vi "archivoaespectro.vi"(5 "data 2":string[][](array[string])) -> (3 "opciones":bool[](array[boolean]), 4 "Control de espejos 3":T5={"Movimiento de spot en y"=0.78, "Movimiento de spot en x"=0.5255, "tipo "=enum."barrido", "yFin"=0.82, "Paso"=0.01, "xFin"=0.5655} {"Movimiento de spot en x" scale=-10.0..10.0; "Movimiento de spot en y" min=-10.0 max=10.0 scale=-10.0..10.0}, 6 "config. Polarizador 2":T4={"pos inic"=0.0, "pos.final"=5.0, "incremento"=1.0, "velocidad"=0.0}, 8 "Config. fotodiodo y potenciometro 2":T2={"tiempo. lect."=300, "num. med"=20, "tiempo. lectura"=0, "average rate"=0, "Readout Config"="POW", "Tipo de Medición"=enum."Lockin", "usar multimetro"=FALSE}, 10 "Config. voltaje y corriente 2":T3 {"Measurement Function (0:Voltage)" items=["Voltage", "Current", "Power"]; "Unit(V)" items=["V", "mV", "kV", "A", "mA"]; "Function(0:Voltage)" items=["Voltage", "Current"]}, 14 "orden":T6(array[ring]), 15 "Control CCD 2":T1={"Numero de lecturas"=0, "tiempo de lectura (ms)"=100, "Exposure"=0.053229, "Valor Gamma"=1.0, "Ganancia"=33, "Opción"=enum."Espectro", "VISA resource name"="", "Enable Strobe (Disabled)"=FALSE} {"Ganancia" min=0 max=100; "Valor Gamma" min=1.0 max=2.2; "Exposure" min=5e-05 max=0.053229})   [LabVIEW 2016]
panel:
  in  "Control CCD":T1={"Numero de lecturas"=0, "tiempo de lectura (ms)"=100, "Exposure"=0.053229, "Valor Gamma"=1.0, "Ganancia"=33, "Opción"=enum."Espectro", "VISA resource name"="", "Enable Strobe (Disabled)"=FALSE} {"Ganancia" min=0 max=100; "Valor Gamma" min=1.0 max=2.2; "Exposure" min=5e-05 max=0.053229}
  in  "Config. fotodiodo y potenciometro":T2={"tiempo. lect."=300, "num. med"=20, "tiempo. lectura"=0, "average rate"=0, "Readout Config"="POW", "Tipo de Medición"=enum."Lockin", "usar multimetro"=FALSE}
  in  "Config. voltaje y corriente":T3 {"Measurement Function (0:Voltage)" items=["Voltage", "Current", "Power"]; "Unit(V)" items=["V", "mV", "kV", "A", "mA"]; "Function(0:Voltage)" items=["Voltage", "Current"]}
  in  "config. Polarizador":T4={"pos inic"=0.0, "pos.final"=5.0, "incremento"=1.0, "velocidad"=0.0}
  in  "Control de espejos 2":T5={"Movimiento de spot en y"=0.78, "Movimiento de spot en x"=0.5255, "tipo "=enum."barrido", "yFin"=0.82, "Paso"=0.01, "xFin"=0.5655} {"Movimiento de spot en x" scale=-10.0..10.0; "Movimiento de spot en y" min=-10.0 max=10.0 scale=-10.0..10.0}
  in  "Array":bool[](array[boolean])=[FALSE, FALSE, FALSE, FALSE, FALSE]
  # "Espectro"
  # "Imágen"
  # "Espectro"
  # "Imágen"
  # "Amplificador Lock in"
  # "potenciometro"
  # "Amplificador Lock in"
  # "potenciometro"
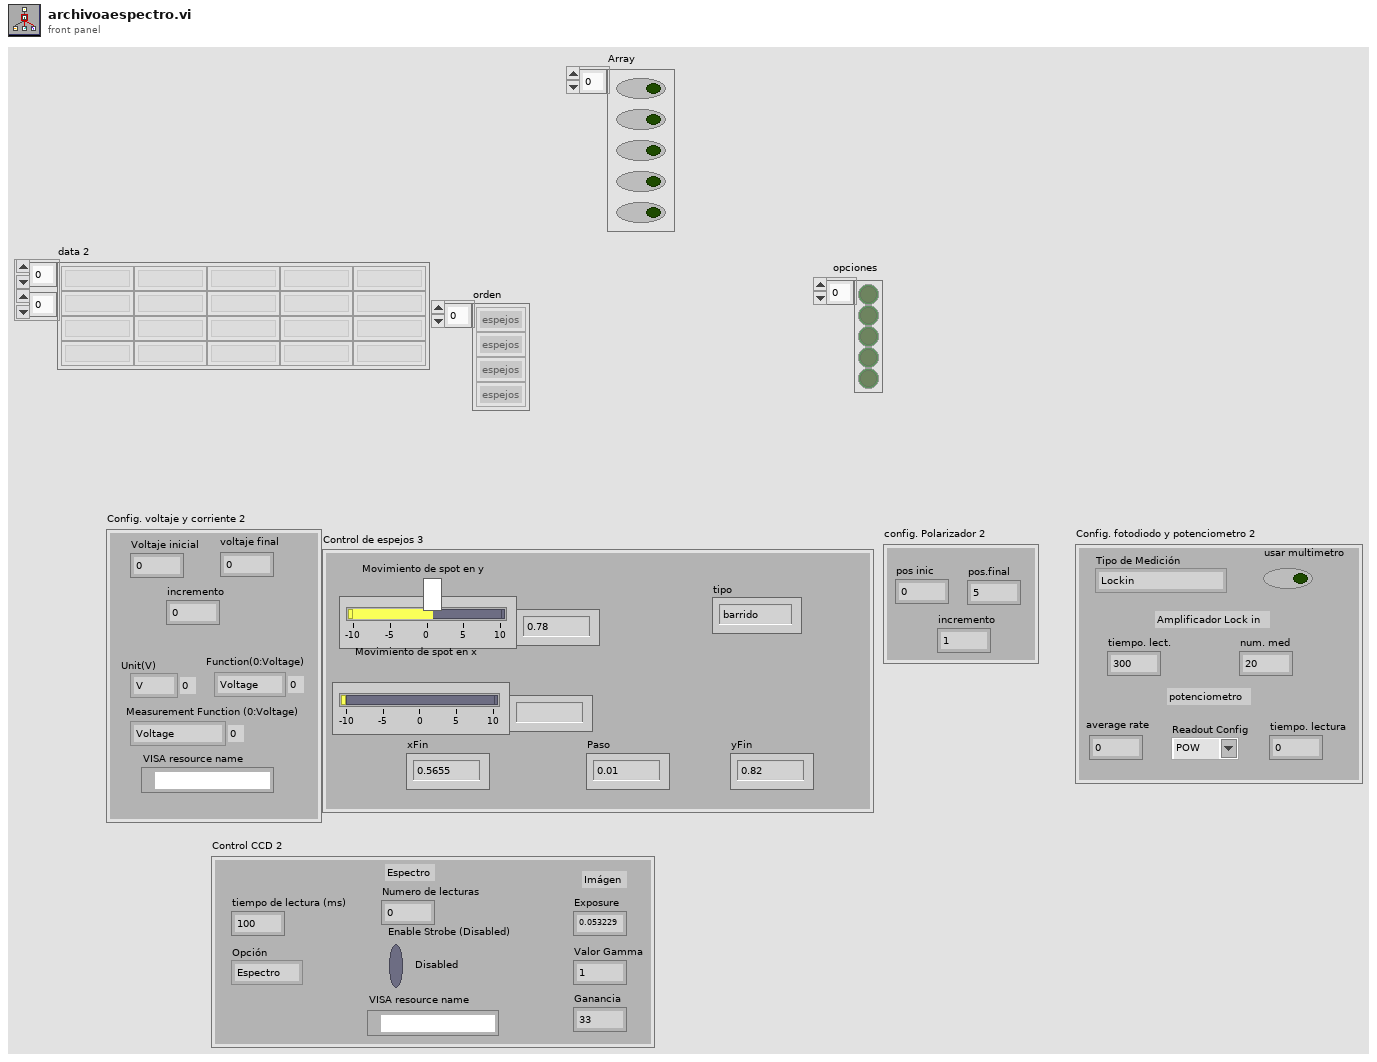
[diagram p1: front panel]
types:
  T1 = cluster{"Numero de lecturas":i32, "tiempo de lectura (ms)":u32, "Exposure":dbl, "Valor Gamma":dbl, "Ganancia":i64, "Opción":enum16{"Espectro", "Imágen"}, "VISA resource name":refnum<visa-resource-name>, "Enable Strobe (Disabled)":bool}
  T2 = cluster{"tiempo. lect.":i32, "num. med":i32, "tiempo. lectura":i32, "average rate":i32, "Readout Config":string, "Tipo de Medición":enum16{"Lockin", "Lockin-potenciometro", "Potenciometro"}, "usar multimetro":bool}
  T3 = cluster{"Voltaje inicial":dbl, "incremento":dbl, " voltaje final":dbl, "Function(0:Voltage)":u16, "Unit(V)":u16, "Measurement Function (0:Voltage)":u16, "VISA resource name":refnum<visa-resource-name>}
  T4 = cluster{"pos inic":dbl, "pos.final":dbl, "incremento":dbl, "velocidad":dbl}
  T5 = cluster{"Movimiento de spot en y":dbl, "Movimiento de spot en x":ext, "tipo ":enum16{"manual", "barrido"}, "yFin":dbl, "Paso":dbl, "xFin":dbl}
  T6 = enum16{"espejos", "polarizador", "voltaje", "potenciometro y lockin", "CCD"}[]
  T7 = enum16{"espejos", "polarizador", "voltaje", "potenciometro y lockin", "CCD"}
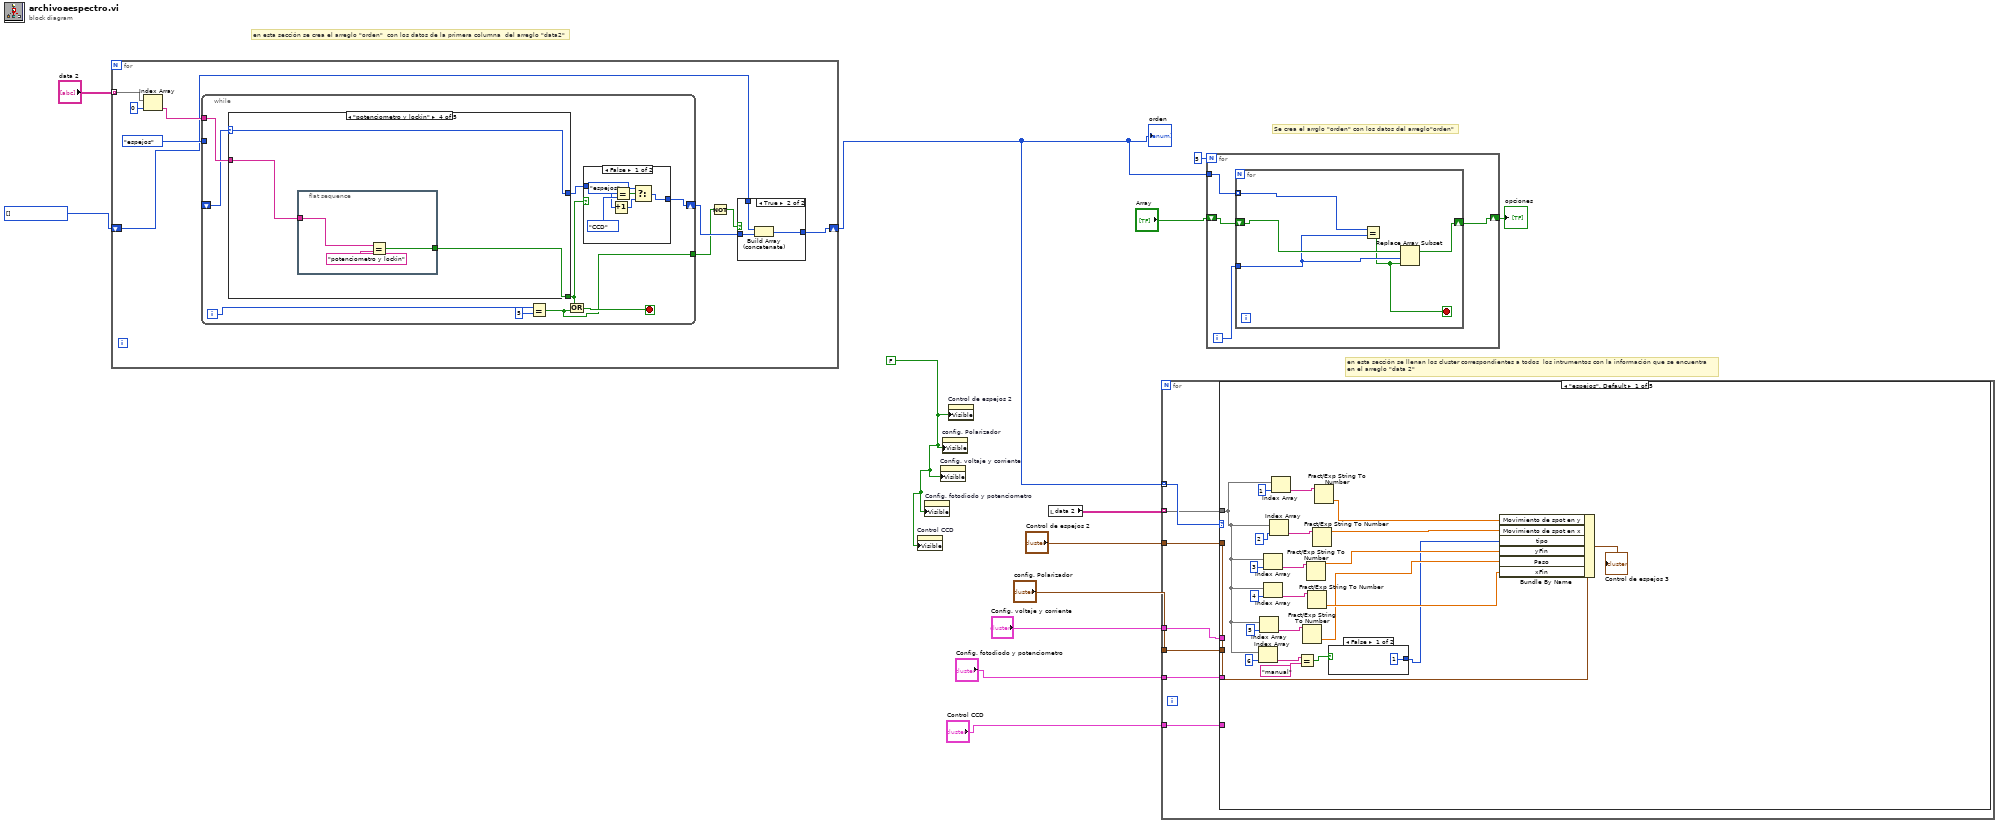
[diagram p0: block diagram]
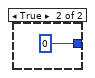
[diagram p2: hidden frame]
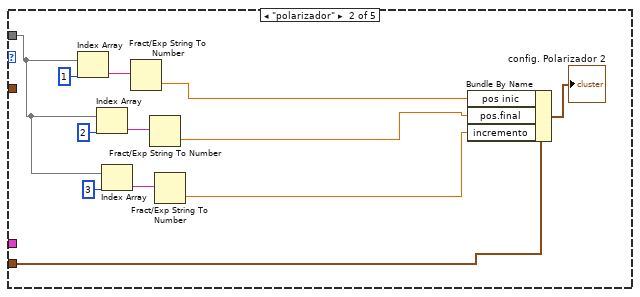
[diagram p3: hidden frame]
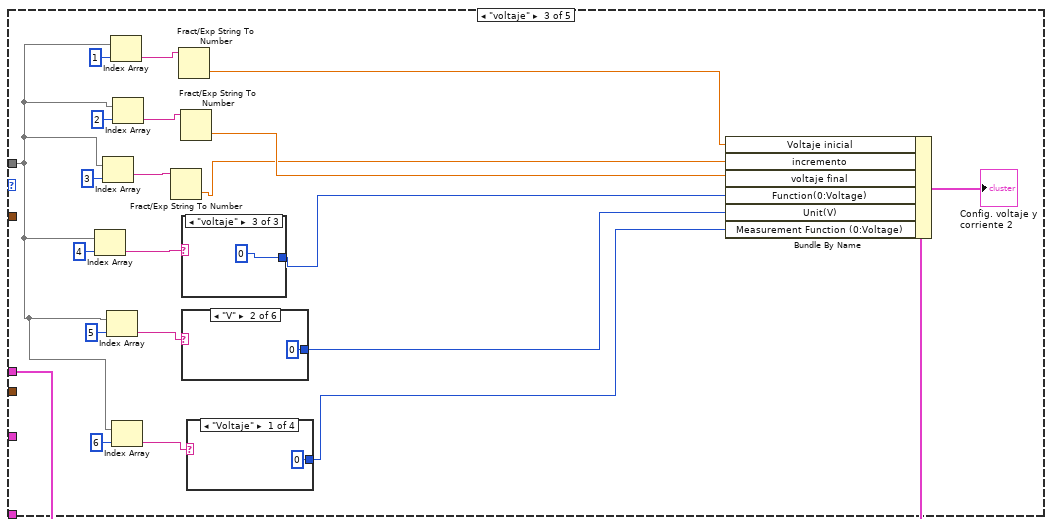
[diagram p4: hidden frame]
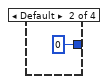
[diagram p5: hidden frame]
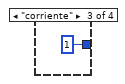
[diagram p6: hidden frame]
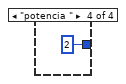
[diagram p7: hidden frame]
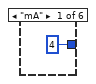
[diagram p8: hidden frame]
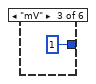
[diagram p9: hidden frame]
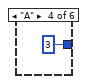
[diagram p10: hidden frame]
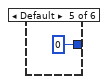
[diagram p11: hidden frame]
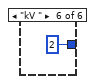
[diagram p12: hidden frame]
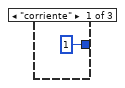
[diagram p13: hidden frame]
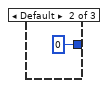
[diagram p14: hidden frame]
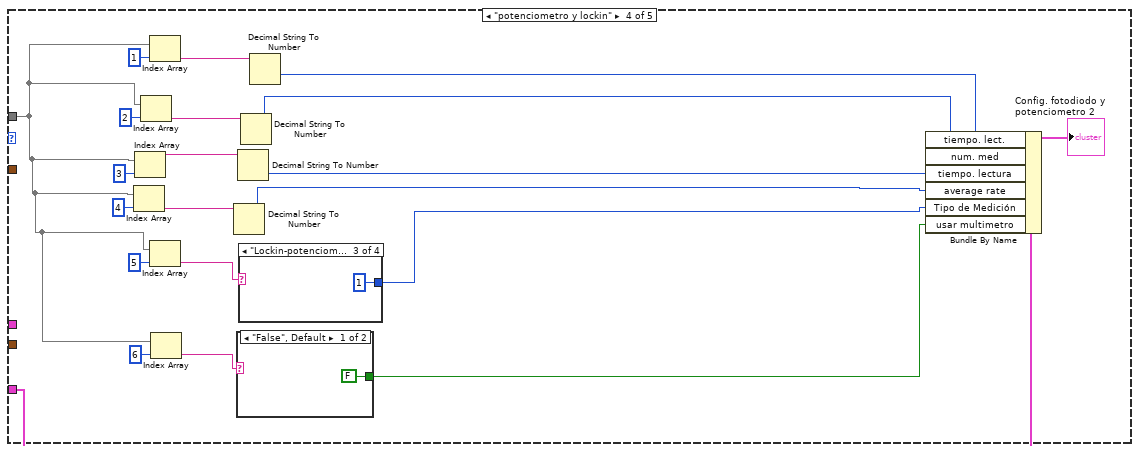
[diagram p15: hidden frame]
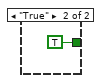
[diagram p16: hidden frame]
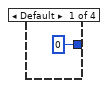
[diagram p17: hidden frame]
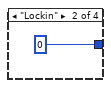
[diagram p18: hidden frame]
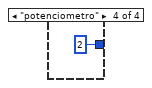
[diagram p19: hidden frame]
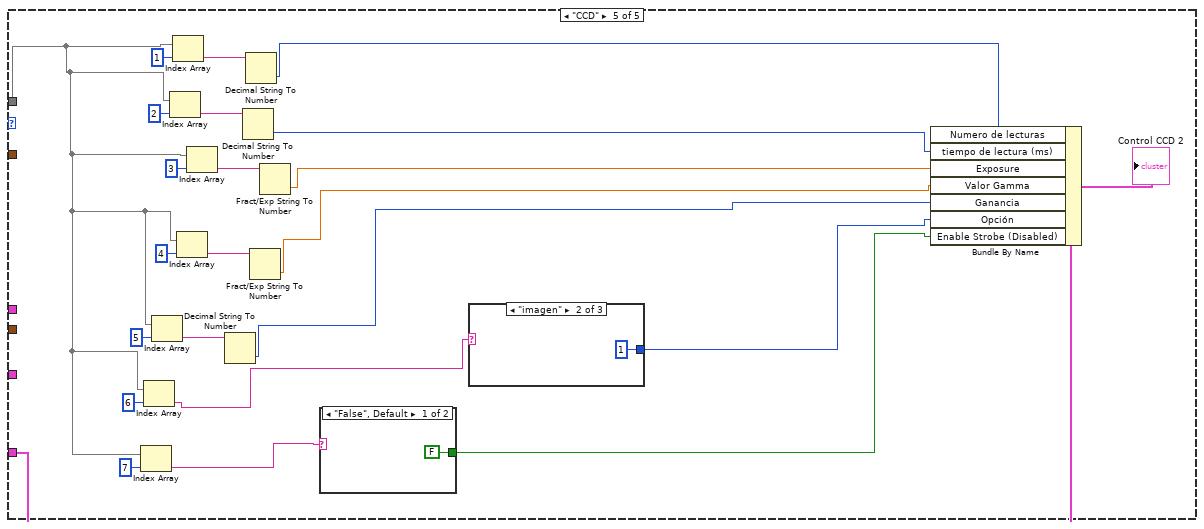
[diagram p20: hidden frame]
diagram:
  w1 = FALSE ("Visible")
  w9 = T6 [] items=["espejos", "polarizador", "voltaje", "potenciometro y lockin", "CCD"] ("Array 3")
  # "en esta sección se llenan los cluster correspondientes a todos  los intrumentos con la información que se encuentra\nen el arreglo \"data 2\""
  # "Se crea el arrglo \"orden\" con los datos del arreglo\"orden\""
  # "en esta sección se crea el arreglo \"orden\"  con los datos de la primera columna  del arreglo \"data2\""
  n1 = for {
    tunnel: "data 2" -> [w22] mode=indexing
    shift-right: [w14] -> w8
    shift-left: w9 -> [w15]
    n2 = Index Array(array=w22, index=0) -> (element=w20:string)
    n3 = while {
      tunnel: w20 -> [w35]
      tunnel: T7."espejos" ("Enum") -> [_]
      shift-right: [w30] -> w18
      shift-left: _ -> [w34]
      tunnel: [w27] -> w16
      i -> [w33]
      stop <- w31 stop-if-true
      n4 = case shown="\"potenciometro y lockin\"" w34 {
        selector: w34 -> [w43 w51 w57 w63 w69]
        tunnel: w35 -> [w45 w49 w56 w62 w68]
        tunnel: [w43 w51 w57 w63 w69] -> w28
        tunnel: [w44 w50 w55 w61 w67] -> w29
        frame "espejos", Default {
          n5 = flat-sequence {
            tunnel: w45 -> [w47]
            tunnel: [w46] -> w44
            frame #0 {
              n6 = Equal?(x=w47, y="espejos") -> (x = y?=w46:bool)
            }
          }
        }
        frame "polarizador" {
          n7 = flat-sequence {
            tunnel: w49 -> [w53]
            tunnel: [w52] -> w50
            frame #0 {
              n8 = Equal?(x=w53, y="polarizador") -> (x = y?=w52:bool)
            }
          }
        }
        frame "voltaje" {
          n9 = flat-sequence {
            tunnel: w56 -> [w59]
            tunnel: [w58] -> w55
            frame #0 {
              n10 = Equal?(x=w59, y="voltaje") -> (x = y?=w58:bool)
            }
          }
        }
        frame "potenciometro y lockin" {
          n11 = flat-sequence {
            tunnel: w62 -> [w65]
            tunnel: [w64] -> w61
            frame #0 {
              n12 = Equal?(x=w65, y="potenciometro y lockin") -> (x = y?=w64:bool)
            }
          }
        }
        frame "CCD" {
          n13 = flat-sequence {
            tunnel: w68 -> [w71]
            tunnel: [w70] -> w67
            frame #0 {
              n14 = Equal?(x=w71, y=" CCD") -> (x = y?=w70:bool)
            }
          }
        }
      }
      n15 = Equal?(x=w33, y=5) -> (x = y?=w27:bool)
      n16 = Or(x=w29, y=w27) -> (x .or. y?=w31:bool)
      n17 = case shown="False" w29 {
        tunnel: [w36 w42] -> w30
        tunnel: w28 -> [w38 w42]
        frame False {
          n18 = Increment(x=w38) -> (x+1=w39:T7)
          n19 = Equal?(x=w38, y=T7."CCD" ("x")) -> (x = y?=w41:bool)
          n20 = Select(t=T7."espejos", s=w41, f=w39) -> (s? t:f=w36:T7)
        }
        frame True {
        }
      }
    }
    n21 = Not(x=w16) -> (.not. x?=w17:bool)
    n22 = case shown="True" w17 {
      tunnel: w15 -> [w23 w26]
      tunnel: w18 -> [_ w25]
      tunnel: [w23 w24] -> w14
      frame False {
      }
      frame True {
        n23 = Build Array (concatenate)(w26, w25) -> (w24:T6)
      }
    }
  }
  "orden" <- w8
  n24 = property on="Control CCD" class="Clust (strict)"("Visible"=w1) -> ()  [unwired: 2 in, 2 out]
  n25 = property on="Config. fotodiodo y potenciometro" class="Clust (strict)"("Visible"=w1) -> ()  [unwired: 2 in, 2 out]
  n26 = property on="Config. voltaje y corriente" class="Clust (strict)"("Visible"=w1) -> ()  [unwired: 2 in, 2 out]
  n27 = property on="config. Polarizador" class="Clust (strict)"("Visible"=w1) -> ()  [unwired: 2 in, 2 out]
  n28 = property on="Control de espejos 2" class="Clust (strict)"("Visible"=w1) -> ()  [unwired: 2 in, 2 out]
  n29 = local read "data 2"() -> (w7:string[][])
  n30 = for {
    tunnel: w8 -> [w79] mode=indexing
    tunnel: w7 -> [w78] mode=indexing
    tunnel: "Control de espejos 2" -> [w77]
    tunnel: "config. Polarizador" -> [w76]
    tunnel: "Config. voltaje y corriente" -> [w75]
    tunnel: "Config. fotodiodo y potenciometro" -> [w74]
    tunnel: "Control CCD" -> [w73]
    n31 = case shown="\"espejos\", Default" w79 {
      tunnel: w78 -> [w86 w106 w118 w154 w184]
      tunnel: w77 -> [w101 _ _ _ _]
      tunnel: w76 -> [_ w115 _ _ _]
      tunnel: w75 -> [_ _ w136 _ _]
      tunnel: w74 -> [_ _ _ w170 _]
      tunnel: w73 -> [_ _ _ _ w200]
      frame "espejos", Default {
        n32 = Index Array(array=w86, index=6) -> (element=w84:string)
        n33 = Index Array(array=w86, index=5) -> (element=w89:string)
        n34 = Index Array(array=w86, index=3) -> (element=w95:string)
        n35 = Index Array(array=w86, index=4) -> (element=w92:string)
        n36 = Index Array(array=w86, index=2) -> (element=w98:string)
        n37 = Index Array(array=w86, index=1) -> (element=w100:string)
        n38 = Equal?(x=w84, y="manual") -> (x = y?=w85:bool)
        n39 = Fract/Exp String To Number(string=w89) -> (number=w88:dbl)  [unwired: 3 in, 1 out]
        n40 = Fract/Exp String To Number(string=w95) -> (number=w94:dbl)  [unwired: 3 in, 1 out]
        n41 = Fract/Exp String To Number(string=w92) -> (number=w91:dbl)  [unwired: 3 in, 1 out]
        n42 = Fract/Exp String To Number(string=w98) -> (number=w97:dbl)  [unwired: 3 in, 1 out]
        n43 = Fract/Exp String To Number(string=w100) -> (number=w99:dbl)  [unwired: 3 in, 1 out]
        n44 = case shown="False" w85 {
          tunnel: [1 0] -> w81
          frame False {
          }
          frame True {
          }
        }
        n45 = Bundle By Name(cluster=w101, "Movimiento de spot en y"=w99, "Movimiento de spot en x"=w97, "tipo"=w81, "yFin"=w94, "Paso"=w88, "xFin"=w91) -> (→"Control de espejos 3":T5)
      }
      frame "polarizador" {
        n46 = Index Array(array=w106, index=1) -> (element=w114:string)
        n47 = Index Array(array=w106, index=2) -> (element=w111:string)
        n48 = Index Array(array=w106, index=3) -> (element=w108:string)
        n49 = Fract/Exp String To Number(string=w114) -> (number=w112:dbl)  [unwired: 3 in, 1 out]
        n50 = Fract/Exp String To Number(string=w111) -> (number=w109:dbl)  [unwired: 3 in, 1 out]
        n51 = Fract/Exp String To Number(string=w108) -> (number=w105:dbl)  [unwired: 3 in, 1 out]
        n52 = Bundle By Name(cluster=w115, "pos inic"=w112, "pos.final"=w109, "incremento"=w105) -> (→"config. Polarizador 2":T4)
      }
      frame "voltaje" {
        n53 = Index Array(array=w118, index=4) -> (element=w125:string)
        n54 = Index Array(array=w118, index=3) -> (element=w129:string)
        n55 = Index Array(array=w118, index=5) -> (element=w122:string)
        n56 = Index Array(array=w118, index=1) -> (element=w135:string)
        n57 = Index Array(array=w118, index=6) -> (element=w119:string)
        n58 = Index Array(array=w118, index=2) -> (element=w132:string)
        n59 = Fract/Exp String To Number(string=w129) -> (number=w127:dbl)  [unwired: 3 in, 1 out]
        n60 = Fract/Exp String To Number(string=w135) -> (number=w134:dbl)  [unwired: 3 in, 1 out]
        n61 = Fract/Exp String To Number(string=w132) -> (number=w130:dbl)  [unwired: 3 in, 1 out]
        n62 = case shown="\"voltaje\"" w125 {
          tunnel: [1 0 0] -> w124
          frame "corriente" {
          }
          frame Default {
          }
          frame "voltaje" {
          }
        }
        n63 = case shown="\"V\"" w122 {
          tunnel: [4 0 1 3 0 2] -> w121
          frame "mA" {
          }
          frame "V" {
          }
          frame "mV" {
          }
          frame "A" {
          }
          frame Default {
          }
          frame "kV " {
          }
        }
        n64 = case shown="\"Voltaje\"" w119 {
          tunnel: [0 0 1 2] -> w117
          frame "Voltaje" {
          }
          frame Default {
          }
          frame "corriente" {
          }
          frame "potencia " {
          }
        }
        n65 = Bundle By Name(cluster=w136, "Voltaje inicial"=w134, "incremento"=w127, "voltaje final"=w130, "Function(0:Voltage)"=w124, "Unit(V)"=w121, "Measurement Function (0:Voltage)"=w117) -> (→"Config. voltaje y corriente 2":T3)
      }
      frame "potenciometro y lockin" {
        n66 = Index Array(array=w154, index=4) -> (element=w160:string)
        n67 = Index Array(array=w154, index=3) -> (element=w163:string)
        n68 = Index Array(array=w154, index=2) -> (element=w166:string)
        n69 = Index Array(array=w154, index=1) -> (element=w169:string)
        n70 = Index Array(array=w154, index=5) -> (element=w156:string)
        n71 = Index Array(array=w154, index=6) -> (element=w152:string)
        n72 = Decimal String To Number(string=w160) -> (number=w158:i32)  [unwired: 2 in, 1 out]
        n73 = case shown="\"False\", Default" w152 {
          tunnel: [FALSE TRUE] -> w151
          frame "False", Default {
          }
          frame "True" {
          }
        }
        n74 = Decimal String To Number(string=w163) -> (number=w161:i32)  [unwired: 2 in, 1 out]
        n75 = case shown="\"Lockin-potenciometro\"" w156 {
          tunnel: [0 0 1 2] -> w155
          frame Default {
          }
          frame "Lockin" {
          }
          frame "Lockin-potenciometro" {
          }
          frame "potenciometro" {
          }
        }
        n76 = Decimal String To Number(string=w166) -> (number=w164:i32)  [unwired: 2 in, 1 out]
        n77 = Decimal String To Number(string=w169) -> (number=w168:i32)  [unwired: 2 in, 1 out]
        n78 = Bundle By Name(cluster=w170, "tiempo. lect."=w168, "num. med"=w164, "tiempo. lectura"=w161, "average rate"=w158, "Tipo de Medición"=w155, "usar multimetro"=w151) -> (→"Config. fotodiodo y potenciometro 2":T2)
      }
      frame "CCD" {
        n79 = Index Array(array=w184, index=7) -> (element=w182:string)
        n80 = Index Array(array=w184, index=6) -> (element=w180:string)
        n81 = Index Array(array=w184, index=5) -> (element=w194:string)
        n82 = Index Array(array=w184, index=2) -> (element=w196:string)
        n83 = Index Array(array=w184, index=1) -> (element=w199:string)
        n84 = Index Array(array=w184, index=4) -> (element=w188:string)
        n85 = Index Array(array=w184, index=3) -> (element=w190:string)
        n86 = Decimal String To Number(string=w194) -> (number=w191:i32)  [unwired: 2 in, 1 out]
        n87 = Decimal String To Number(string=w196) -> (number=w178:i32)  [unwired: 2 in, 1 out]
        n88 = Decimal String To Number(string=w199) -> (number=w198:i32)  [unwired: 2 in, 1 out]
        n89 = Fract/Exp String To Number(string=w188) -> (number=w185:dbl)  [unwired: 3 in, 1 out]
        n90 = Fract/Exp String To Number(string=w190) -> (number=w186:dbl)  [unwired: 3 in, 1 out]
        n91 = case shown="\"False\", Default" w182 {
          tunnel: [FALSE TRUE] -> w181
          frame "False", Default {
          }
          frame "True" {
          }
        }
        n92 = case shown="\"imagen\"" w180 {
          tunnel: [0 1 0] -> w179
          frame Default {
          }
          frame "imagen" {
          }
          frame "espectro" {
          }
        }
        n93 = Bundle By Name(cluster=w200, "Numero de lecturas"=w198, "tiempo de lectura (ms)"=w178, "Exposure"=w186, "Valor Gamma"=w185, "Ganancia"=w191, "Opción"=w179, "Enable Strobe (Disabled)"=w181) -> (→"Control CCD 2":T1)
      }
    }
  }
  n94 = for {
    N: 5 -> [_]
    tunnel: w8 -> [w210]
    shift-right: [w208] -> w11
    shift-left: "Array" -> [w209]
    i -> [w207]
    n95 = for {
      tunnel: w210 -> [w215] mode=indexing
      shift-right: [w213] -> w208
      shift-left: w209 -> [w214]
      tunnel: w207 -> [w212]
      stop <- w211 stop-if-true
      n96 = Equal?(x=w215, y=w212) -> (x = y?=w211:bool)
      n97 = Replace Array Subset(array=w214, new element=w211, index=w212) -> (w213:bool[])
    }
  }
  "opciones" <- w11
